vi "GUI.vi"() -> ()   [LabVIEW 2023]
uses:
  <vilib>/Instr/_visa.llb/VISA Configure Serial Port (Instr).vi
  <vilib>/addons/database/Connection.llb/DB Tools Open Connec (String).vi
  <vilib>/addons/database/Connection.llb/Conn Execute.vi
  <vilib>/addons/database/Recordset.llb/Rec Destroy - Connection.vi
  <vilib>/addons/database/NI_Database_API.lvlib
panel:
  out "Waveform Graph 2":dbl[](graph)
  in  "stop 2":bool
  out "concatenated string":string
  in  "Unidades":string(combo)
  in  "Canal":enum32{"Item 0", "Item 1"}(radio)
  in  "Guardar":bool
  in  "Autor":string
  out "index":dbl
  out "InicialArr":dbl[](array[numeric])
  out "value":dbl
  out "Canal1":bool
  out "Canal2":bool
  in  "VISA resource name":refnum<visa-resource-name>
  in  "stop":bool
  in  "10 V":bool
  in  "5 V":bool
  in  "2.5 V":bool
  in  "1 V":bool
  in  "10 mV":bool
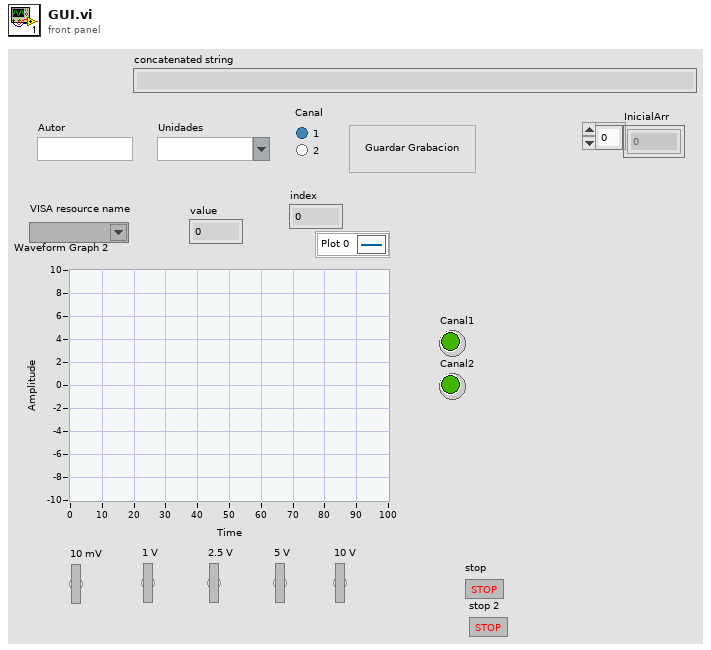
[diagram p1: front panel]
types:
  T1 = typedef "NI_Database_API.lvlib/Conn ObjectReference.ctl" = refnum<k1>
  T2 = typedef "NI_Database_API.lvlib/Rec ObjectReference.ctl" = refnum<k1>
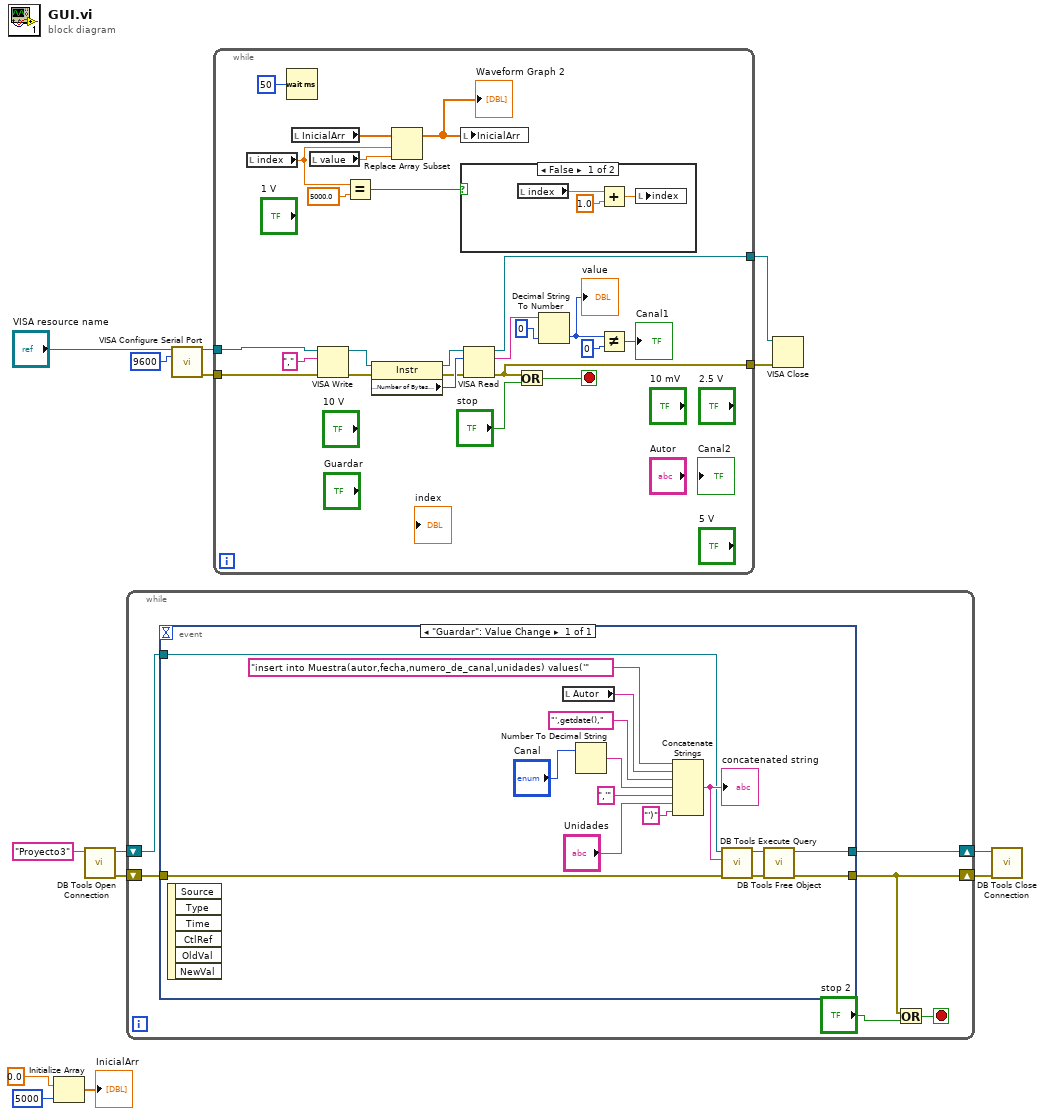
[diagram p0: block diagram]
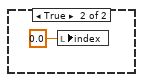
[diagram p2: hidden frame]
diagram:
  n1 = Initialize Array(0.0 ("element"), 5000 ("dimension size")) -> (→"InicialArr":dbl[])
  n2 = call-poly <vilib>:"DB Tools Open Connection.vi"("connection information"="Proyecto3") -> ("error out"=w4:errorcluster, "connection reference"=w3:T1)  [unwired: 7 in]
  n3 = while {
    shift-right: [w16] -> w2
    shift-left: w4 -> [w20]
    shift-right: [w18] -> w1
    shift-left: w3 -> [w19]
    stop <- w17 stop-if-true
    n4 = event shown="[0] \"Guardar\": Value Change" {
      selector: _ -> [_]
      dyn-events: _ -> [_]
      timeout: _ -> [_]
      tunnel: [w24] -> w16
      tunnel: [w23] -> w18
      tunnel: w20 -> [w22]
      tunnel: w19 -> [w21]
      event "Guardar": Value Change {
        n5 = event-data() -> ()  [unwired: 1 in, 6 out]
        n6 = local read "Autor"() -> (w32:string)
        n7 = Number To Decimal String(number="Canal") -> (decimal integer string=w34:string)  [unwired: 1 in]
        n8 = Concatenate Strings("insert into Muestra(autor,fecha,numero_de_canal,unidades) values('", w32, "',getdate(),", w34, ",'" ("string"), "Unidades", "')" ("string")) -> (w35:string)
        "concatenated string" <- w35
        n9 = call-poly <vilib>:"DB Tools Execute Query.vi"("error in (no error)"=w22, "SQL query"=w35, "connection reference"=w21) -> ("error out"=w25:errorcluster, "recordset reference"=w26:T2)  [unwired: 5 in]
        n10 = call-poly <vilib>:"DB Tools Free Object.vi"("error in (no error)"=w25, "recordset reference"=w26) -> ("error out"=w24:errorcluster, "connection reference"=w23:T1)  [unwired: 8 in]
      }
    }
    n11 = Or(x=w16, y="stop 2") -> (x .or. y?=w17:bool)
  }
  n12 = call-poly "VISA Configure Serial Port"("VISA resource name"="VISA resource name", "baud rate (9600)"=u32 9600) -> ("VISA resource name out"=w14:refnum<visa-resource-name>, "error out"=w11:errorcluster)  [unwired: 12 in]
  n13 = while {
    tunnel: w14 -> [w55]
    tunnel: [w48] -> w13
    tunnel: [w49] -> w12
    tunnel: w11 -> [w53]
    stop <- w37 stop-if-true
    n14 = local read "index"() -> (w43:dbl)
    n15 = Wait (ms)(milliseconds to wait=u32 50) -> ()  [unwired: 1 out]
    n16 = local read "InicialArr"() -> (w42:dbl[])
    n17 = local read "value"() -> (w41:dbl)
    n18 = VISA Write(VISA resource name=w55, write buffer=",", error in (no error)=w53) -> (VISA resource name out=w57:refnum<visa-resource-name>, error out=w52:errorcluster)  [unwired: 1 out]
    n19 = Equal?(x=w43, y=5000.0) -> (x = y?=w44:bool)
    n20 = property class="Instr"(reference=w57, error in=w52) -> (reference out=w56:refnum<visa-resource-name>, error out=w50:errorcluster, "Serial Settings:Number of Bytes at Serial Port"=w51:u32)
    n21 = Replace Array Subset(array=w42, new element=w41, index=w43) -> (w36:dbl[])
    "Waveform Graph 2" <- w36
    n22 = local write "InicialArr"(w36) -> ()
    n23 = case shown="False" w44 {
      frame False {
        n24 = local read "index"() -> (w60:dbl)
        n25 = Add(x=w60, y=1.0 ("index")) -> (x+y=w61:dbl)
        n26 = local write "index"(w61) -> ()
      }
      frame True {
        n27 = local write "index"(0.0 ("index")) -> ()
      }
    }
    n28 = VISA Read(VISA resource name=w56, byte count=w51, error in (no error)=w50) -> (VISA resource name out=w48:refnum<visa-resource-name>, read buffer=w47:string, error out=w49:errorcluster)  [unwired: 1 out]
    n29 = Or(x=w49, y="stop") -> (x .or. y?=w37:bool)
    n30 = Decimal String To Number(string=w47, default (0L)=0 ("default (0 I32)")) -> (number=w40:i32)  [unwired: 1 in, 1 out]
    "value" <- w40
    n31 = Not Equal?(x=w40, y=0) -> (x != y?=→"Canal1":bool)
  }
  n32 = VISA Close(VISA resource name=w13, error in (no error)=w12) -> ()  [unwired: 1 out]
  n33 = call <vilib>:"DB Tools Close Connection.vi"("error in (no error)"=w2, "connection reference"=w1) -> ()  [unwired: 5 in, 1 out]
